vi "2023 actual arm.vi"(8 "y (final pt)":dbl, 9 "x (final pt)":dbl, 10 "length 2nd arm":dbl, 11 "length 1st arm":dbl) -> (0 "y1c2 (1st arm)":dbl, 1 "x1c2 (1st arm)":dbl, 2 "y1c1 (1st arm)":dbl, 3 "x1c1 (1st arm)":dbl)   [LabVIEW 2023]
panel:
  out "p1 (for debug":dbl
  out "q2 (config 1)":dbl
  out "q2 (config 2)":dbl
  out "q1 (config 2)":dbl
  out "x1c2 (2nd arm)":dbl
  out "y1c2 (2nd arm)":dbl
  out "y1c1 (2nd arm)":dbl
  out "x1c1 (2nd arm)":dbl
  out "q1 (config 1)":dbl
  out "a2 (for debug)":dbl
  out "Configuration 2":cluster{"X":dbl, "Y":dbl}[](graph)
  out "Configuration 1":cluster{"X":dbl, "Y":dbl}[](graph)
  out "2nd absolute angle":dbl
  out "neg relative angle":dbl
  out "XY Graph 2":cluster{"X":dbl, "Y":dbl}[](graph)
  out "XY Graph":cluster{"X":dbl, "Y":dbl}[](graph)
  out "pos absolute angle":dbl
  out "relative angle":dbl
  in  "upper arm length":dbl
  in  "lower arm length":dbl
  in  "y":dbl
  in  "x":dbl
  # "bugs:\n(-2, 1) --> (2, -1) NO WORK!\n(2, -1) --> (2, -1) WORKS!\n(-3, 0) --> (3, 0) NO WORK!\n(4, 0) --> (4, 0) WORKS! \n\nsolution:\nif x is negative --> flip final x (:"
  # "angles (q's) in radians"
  # "Bugs I've Found (6/27): \n - neg X pos Y is wrong (fixed: 8/1/23) \n - X can't be 0 or else code breaks (#dealwithit)\n\n Next Steps After Killing Bugs *spray sounds*:\n - Don't let user type negative Y values (or else... bye bye 2DOF)"
  # "fix goofy ahh overlap"
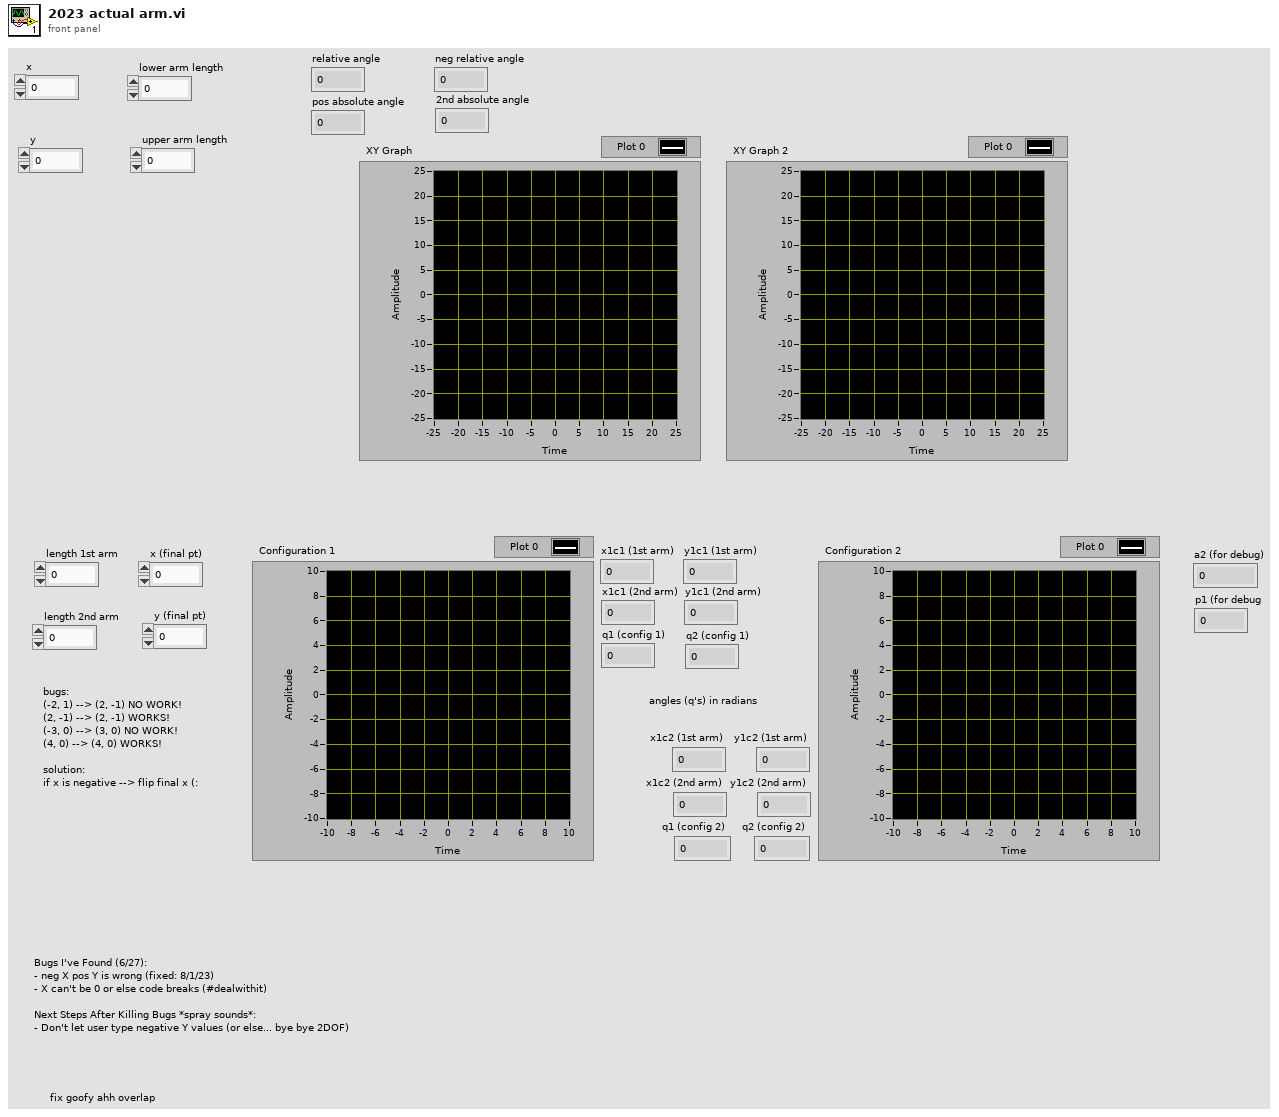
[diagram p1: front panel]
types:
  T1 = cluster{"x1 graph (2nd arm)":dbl, "y1 graph (2nd arm)":dbl}
  T2 = cluster{"x1 graph (2nd arm)":dbl, "y1 graph (2nd arm)":dbl}[]
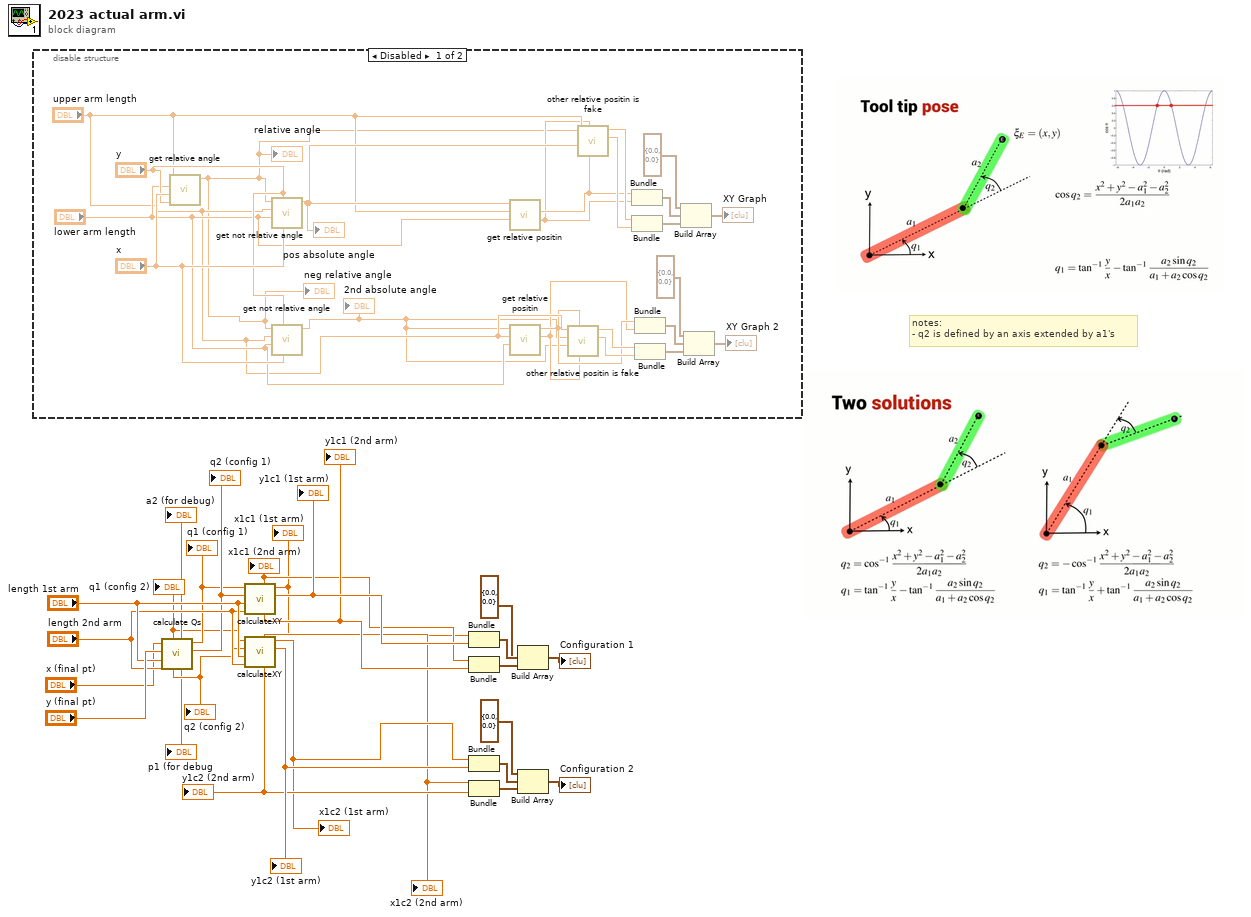
[diagram p0: block diagram]
diagram:
  # "notes:\n- q2 is defined by an axis extended by a1's"
  n1 = disable-structure shown="Disabled" {
    frame Disabled {
      n2 = call "get relative angle.vi"("y"="y", "x"="x", "lower arm length"="lower arm length", "upper arm length"="upper arm length") -> ("arccos(x)"=w28:dbl)  [unwired: 7 in]
      "relative angle" <- w28
      "neg relative angle" <- w28
      n3 = call "get not relative angle.vi"("x"="x", "y"="y", "lower arm length"="lower arm length", "upper arm length"="upper arm length", "arccos(x)"=w28) -> ("Numeric"=w43:dbl)  [unwired: 6 in]
      "pos absolute angle" <- w43
      n4 = call "get not relative angle.vi"("x"="x", "y"="y", "lower arm length"="lower arm length", "upper arm length"="upper arm length", "arccos(x)"=w28) -> ("Numeric"=w27:dbl)  [unwired: 6 in]
      "2nd absolute angle" <- w27
      n5 = call "get relative positin.vi"("lower arm length"="lower arm length", "upper arm length"="upper arm length", "theta"=w43) -> ("x"=w32:dbl, "y"=w31:dbl)  [unwired: 7 in]
      n6 = call "get relative positin.vi"("lower arm length"="lower arm length", "upper arm length"="upper arm length", "theta"=w27) -> ("x"=w29:dbl, "y"=w30:dbl)  [unwired: 7 in]
      n7 = call "other relative positin is fake.vi"("absolute joint y"=w29, "absolute joint x"=w30, "absolute angle"=w27, "arccos(x)"=w27, "upper arm length"="upper arm length") -> ("y"=w36:dbl, "x"=w35:dbl)  [unwired: 5 in]
      n8 = call "other relative positin is fake.vi"("absolute joint y"=w32, "absolute joint x"=w31, "absolute angle"=w43, "arccos(x)"=w28, "upper arm length"="upper arm length") -> ("y"=w49:dbl, "x"=w48:dbl)  [unwired: 5 in]
      n9 = Bundle("x"=w32, "y"=w31) -> (w47:cluster{"x":dbl, "y":dbl})  [unwired: 1 in]
      n10 = Bundle("x"=w48, "y"=w49) -> (w46:cluster{"x":dbl, "y":dbl})  [unwired: 1 in]
      n11 = Bundle("y"=w30, "x"=w29) -> (w33:cluster{"y":dbl, "x":dbl})  [unwired: 1 in]
      n12 = Bundle("x"=w35, "y"=w36) -> (w41:cluster{"x":dbl, "y":dbl})  [unwired: 1 in]
      n13 = Build Array(cluster{dbl, dbl} {0.0, 0.0} ("element"), w47, w46) -> (→"XY Graph":cluster{"x":dbl, "y":dbl}[])
      n14 = Build Array(cluster{dbl, dbl} {0.0, 0.0} ("element"), w33, w41) -> (→"XY Graph 2":cluster{"x":dbl, "y":dbl}[])
    }
    frame Enabled {
    }
  }
  n15 = call "calculate Qs.vi"("length 2"="length 2nd arm", "length 1"="length 1st arm", "y"="y (final pt)", "x"="x (final pt)") -> ("q2 (config 1)"=w11:dbl, "q1 (config 1)"=w9:dbl, "p1 (for debug"=→"p1 (for debug":dbl, "a2 (for debug)"=→"a2 (for debug)":dbl, "q2 (config 2)"=w12:dbl, "q1 (config 2)"=w8:dbl)  [unwired: 2 out]
  "q1 (config 1)" <- w9
  "q1 (config 2)" <- w8
  "q2 (config 2)" <- w12
  "q2 (config 1)" <- w11
  n16 = call "calculateXY.vi"("q1"=w9, "q2"=w11, "length 1"="length 1st arm", "length 2"="length 2nd arm") -> ("x1 graph (2nd arm)"=w6:dbl, "y1 graph (2nd arm)"=w23:dbl, "x1 (1st arm)"=w1:dbl, "y1 (1st arm)"=w25:dbl)  [unwired: 1 in, 2 out]
  "x1c1 (2nd arm)" <- w6
  "x1c1 (1st arm)" <- w1
  "y1c1 (1st arm)" <- w25
  "y1c1 (2nd arm)" <- w23
  n17 = call "calculateXY.vi"("q1"=w8, "q2"=w12, "length 1"="length 1st arm", "length 2"="length 2nd arm") -> ("x1 graph (2nd arm)"=w2:dbl, "y1 graph (2nd arm)"=w16:dbl, "x1 (1st arm)"=w5:dbl, "y1 (1st arm)"=w17:dbl)  [unwired: 1 in, 2 out]
  "x1c2 (1st arm)" <- w5
  "y1c2 (1st arm)" <- w17
  "y1c2 (2nd arm)" <- w16
  "x1c2 (2nd arm)" <- w2
  n18 = Bundle("x1 (1st arm)"=w1, "y1 (1st arm)"=w25) -> (w24:cluster{"x1 (1st arm)":dbl, "y1 (1st arm)":dbl})  [unwired: 1 in]
  n19 = Bundle("x1 graph (2nd arm)"=w6, "y1 graph (2nd arm)"=w23) -> (w22:T1)  [unwired: 1 in]
  n20 = Bundle("x1 (1st arm)"=w5, "y1 (1st arm)"=w17) -> (w19:cluster{"x1 (1st arm)":dbl, "y1 (1st arm)":dbl})  [unwired: 1 in]
  n21 = Bundle("x1 graph (2nd arm)"=w2, "y1 graph (2nd arm)"=w16) -> (w3:T1)  [unwired: 1 in]
  n22 = Build Array(cluster{dbl, dbl} {0.0, 0.0} ("element"), w24, w22) -> (→"Configuration 1":T2)
  n23 = Build Array(cluster{dbl, dbl} {0.0, 0.0} ("element"), w19, w3) -> (→"Configuration 2":T2)
